vi "Post Pelletron Tick.vi"(8 "error in (no error)":errorcluster, 9 "Pelletron data":T1, 11 "Database.lvlib:Data Store.lvclass":refnum<class "Data Store.lvclass">) -> (0 "error out":errorcluster, 3 "Database.lvlib:Data Store.lvclass 2":refnum<class "Data Store.lvclass">)   [LabVIEW 2012, in "Database.lvlib" / "Data Store.lvclass"]
uses:
  Data Store.lvclass
  interface/Pelletron.ctl
  Data Store.lvclass/Data Store.ctl
  <vilib>/addons/database/NI_Database_API.lvlib
  interface/Interface.lvlib
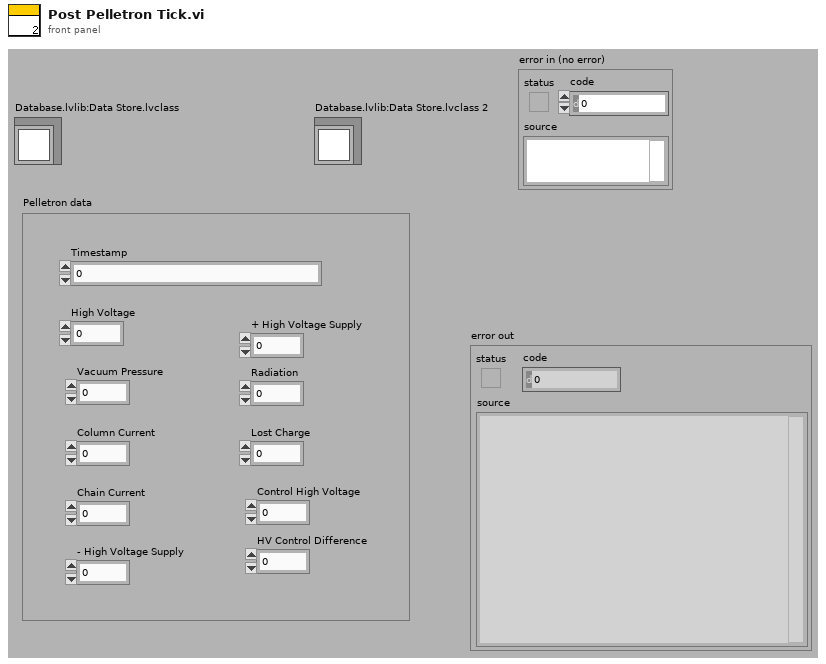
[diagram p1: front panel]
types:
  T1 = typedef "Interface.lvlib/Pelletron.ctl" = cluster{"Timestamp":u64, "High Voltage":sgl, "Vacuum Pressure":sgl, "Column Current":sgl, "Chain Current":sgl, "- High Voltage Supply":dbl, "+ High Voltage Supply":dbl, "Radiation":dbl, "Lost Charge":dbl, "Control High Voltage":dbl, "HV Control Difference":dbl}
  T2 = typedef "NI_Database_API.lvlib/Conn ObjectReference.ctl" = refnum<k1>
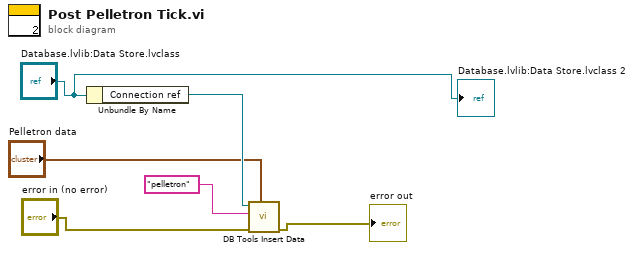
[diagram p0: block diagram]
diagram:
  n1 = Unbundle By Name("Database.lvlib:Data Store.lvclass") -> ("Connection ref"=w6:T2)
  n2 = call <vilib>:"DB Tools Insert Data.vi"("data"="Pelletron data", "error in (no error)"="error in (no error)", "table"="pelletron", "connection reference"=w6) -> ("error out"=→"error out":errorcluster)  [unwired: 6 in, 1 out]
  "Database.lvlib:Data Store.lvclass 2" <- "Database.lvlib:Data Store.lvclass"
